vi "ex_4_1.vi"() -> ()   [LabVIEW 2020]
panel:
  out "Array 3":i32[][](array[numeric])
  out "Array 2":u32[][](array[numeric])
  out "Array":u32[][](array[numeric])
  in  "True = 3x5,\nFalse = 5x3.":bool=TRUE
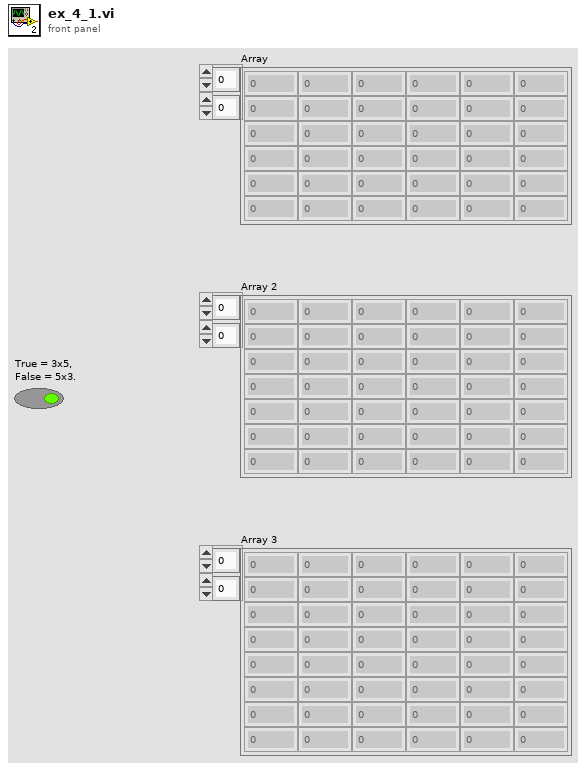
[diagram p1: front panel]
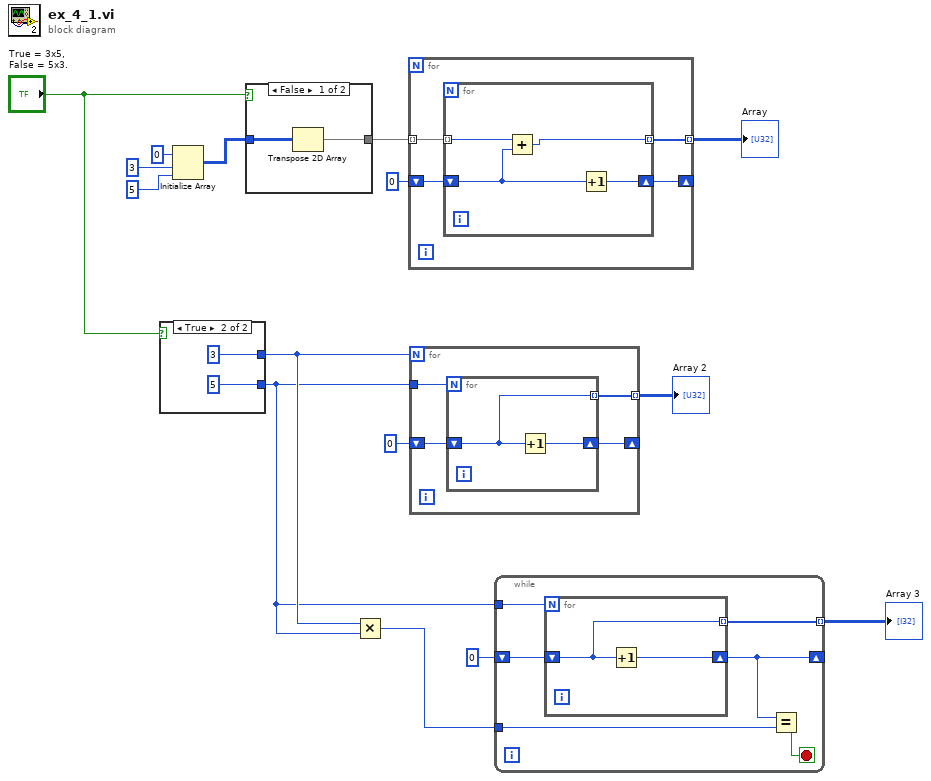
[diagram p0: block diagram]
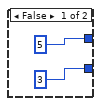
[diagram p2: hidden frame]
diagram:
  n1 = case shown="True" "True = 3x5,\nFalse = 5x3." {
    tunnel: [5 3] -> w2
    tunnel: [3 5] -> w1
    frame False {
    }
    frame True {
    }
  }
  n2 = Initialize Array(u32 0 ("element"), 3 ("dimension size"), 5 ("dimension size")) -> (w12:u32[][])
  n3 = case shown="False" "True = 3x5,\nFalse = 5x3." {
    tunnel: w12 -> [w21 w22]
    tunnel: [w20 w22] -> w11
    frame False {
      n4 = Transpose 2D Array(2D array=w21) -> (transposed array=w20:u32[][])
    }
    frame True {
    }
  }
  n5 = Multiply(x=w2, y=w1) -> (x*y=w3:i32)
  n6 = for {
    tunnel: w11 -> [w26] mode=indexing
    tunnel: [w25] -> w10 mode=indexing
    shift-right: [w23] -> _
    shift-left: u32 0 -> [w24]
    n7 = for {
      tunnel: w26 -> [w29] mode=indexing
      tunnel: [w27] -> w25 mode=indexing
      shift-right: [w30] -> w23
      shift-left: w24 -> [w28]
      n8 = Add(x=w29, y=w28) -> (x+y=w27:u32)
      n9 = Increment(x=w28) -> (x+1=w30:u32)
    }
  }
  "Array" <- w10
  n10 = for {
    N: w2 -> [_]
    tunnel: w1 -> [w34]
    shift-right: [w32] -> _
    shift-left: u32 0 -> [w33]
    tunnel: [w31] -> w7 mode=indexing
    n11 = for {
      N: w34 -> [_]
      shift-right: [w36] -> w32
      shift-left: w33 -> [w35]
      tunnel: [w35] -> w31 mode=indexing
      n12 = Increment(x=w35) -> (x+1=w36:u32)
    }
  }
  "Array 2" <- w7
  n13 = while {
    shift-right: [w39] -> _
    shift-left: 0 -> [w42]
    tunnel: [w41] -> w4 mode=indexing
    tunnel: w3 -> [w40]
    tunnel: w1 -> [w37]
    stop <- w38 stop-if-true
    n14 = for {
      N: w37 -> [_]
      shift-right: [w43] -> w39
      shift-left: w42 -> [w44]
      tunnel: [w44] -> w41 mode=indexing
      n15 = Increment(x=w44) -> (x+1=w43:i32)
    }
    n16 = Equal?(x=w39, y=w40) -> (x = y?=w38:bool)
  }
  "Array 3" <- w4
